vi "string_to_byte_array.vi"(8 "error in (no error)":errorcluster, 10 "Byte":string) -> (0 "error out":errorcluster, 2 "Int array":u8[](array[numeric]))   [LabVIEW 2018]
doc: "Convert an IC6 response string representing a concetenated list of unsigned 1 byte integers into an array of LabVIEW U8."
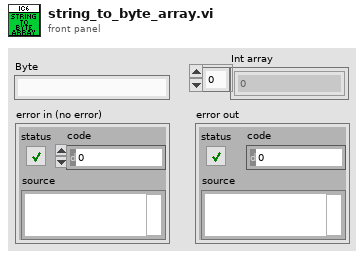
[diagram p1: front panel]
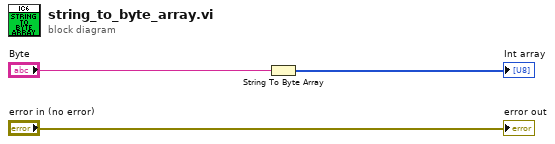
[diagram p0: block diagram]
diagram:
  n1 = String To Byte Array(string="Byte") -> (unsigned byte array=→"Int array":u8[])
  "error out" <- "error in (no error)"
